vi "TipPosition.vi"(8 "error in":errorcluster) -> (0 "error out":errorcluster, 2 "CursorPosition":cluster{dbl, dbl})   [LabVIEW 2016]
uses:
  controls/Enum.ctl
  <vilib>/Utility/error.llb/Error Cluster From Error Code.vi
  <vilib>/rvi/errors/niLvFpgaAdjustHostInterfaceError.vi
  <vilib>/rvi/interface/nirviReadWriteControl/nirviReadWriteControl.xnode
  controls/FPGAVIreferenceTypeDefScanEngine.ctl
  FPGA Bitfiles/qnmController797_usbRIO_controllerFPGAmu.lvbitx
  NiFpgaLv.dll
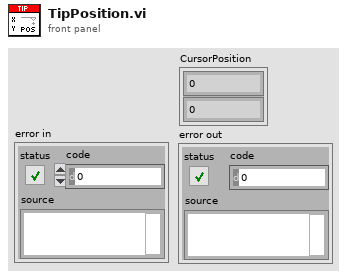
[diagram p1: front panel]
types:
  T1 = typedef "Enum.ctl" = enum16{"Init", "Read", "Write"}
  T2 = cluster{"Width":dbl, "Height":dbl, "X Offset":dbl, "Y Offset":dbl, "Angle":dbl, "Pixels/Line":u16, "Lines":u16, "Time/Line":dbl, "Scan Rate":dbl}
  T3 = cluster{"calibName":string[], "calibParameters":cluster{"Sensitivity":cluster{"Sens X":dbl, "Sens Y":dbl, "Sens Z":dbl}, "Range":cluster{"Range X":dbl, "Range Y":dbl, "Range Z":dbl}, "HV gain":cluster{"HV gain X":dbl, "HV gain Y":dbl, "HV gain Z":dbl}}[], "calibIndex":i32}
  T4 = typedef "FPGAVIreferenceTypeDefScanEngine.ctl" = refnum<k20>
  T5 = cluster{"Sensitivity":cluster{"Sens X":dbl, "Sens Y":dbl, "Sens Z":dbl}, "Range":cluster{"Range X":dbl, "Range Y":dbl, "Range Z":dbl}, "HV gain":cluster{"HV gain X":dbl, "HV gain Y":dbl, "HV gain Z":dbl}}[]
  T6 = cluster{"xOut":fxp<+/-,18,2>, "yOut":fxp<+/-,18,2>}
  T7 = cluster{"Sensitivity":cluster{"Sens X":dbl, "Sens Y":dbl, "Sens Z":dbl}, "Range":cluster{"Range X":dbl, "Range Y":dbl, "Range Z":dbl}, "HV gain":cluster{"HV gain X":dbl, "HV gain Y":dbl, "HV gain Z":dbl}}
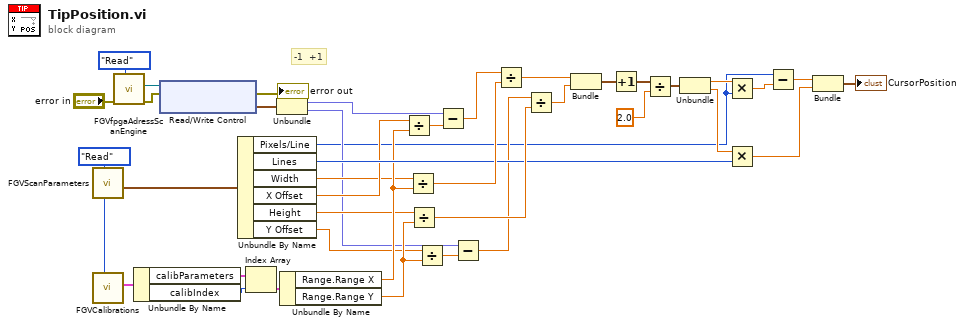
[diagram p0: block diagram]
diagram:
  w36 = Enum."Read" ("Enum")
  # "-1  +1"
  n1 = call "FGVScanParameters.vi"("Enum"=w36) -> ("Scan Parameters Out"=w35:T2)  [unwired: 9 in, 1 out]
  n2 = call "FGVCalibrations.vi"("Enum"=w36) -> ("calibOut"=w37:T3)  [unwired: 9 in, 1 out]
  n3 = call "FGVfpgaAdressScanEngine.vi"("Enum"=Enum."Read", "error in"="error in") -> ("error out"=w34:errorcluster, "FPGA.SEout"=w32:T4)  [unwired: 5 in, 3 out]
  n4 = Unbundle By Name(w37) -> ("calibParameters"=w38:T5, "calibIndex"=w39:i32)
  n5 = xnode "Read/Write Control"("FPGA VI Reference In"=w32, "error in"=w34) -> ("error out"=→"error out":errorcluster, "se.mot.s.origin"=w29:T6)  [unwired: 1 out]
  n6 = Unbundle By Name(w35) -> ("Pixels/Line"=w3:u16, "Lines"=w17:u16, "Width"=w10:dbl, "X Offset"=w13:dbl, "Height"=w9:dbl, "Y Offset"=w7:dbl)
  n7 = Index Array(array=w38, index=w39) -> (element=w40:T7)
  n8 = Unbundle(w29) -> ("xOut"=w12:fxp<+/-,18,2>, "yOut"=w6:fxp<+/-,18,2>)
  n9 = Unbundle By Name(w40) -> ("Range.Range X"=w14:dbl, "Range.Range Y"=w8:dbl)
  n10 = Divide(x=w13, y=w14) -> (x/y=w15:dbl)
  n11 = Divide(x=w10, y=w14) -> (x/y=w28:dbl)
  n12 = Divide(x=w9, y=w8) -> (x/y=w27:dbl)
  n13 = Divide(x=w7, y=w8) -> (x/y=w5:dbl)
  n14 = Subtract(x=w12, y=w15) -> (x-y=w11:dbl)
  n15 = Subtract(x=w6, y=w5) -> (x-y=w4:dbl)
  n16 = Divide(x=w11, y=w28) -> (x/y=w26:dbl)
  n17 = Divide(x=w4, y=w27) -> (x/y=w25:dbl)
  n18 = Bundle(w26, w25) -> (w24:cluster{dbl, dbl})  [unwired: 1 in]
  n19 = Increment(x=w24) -> (x+1=w23:cluster{dbl, dbl})
  n20 = Divide(x=w23, y=2.0) -> (x/y=w20:cluster{dbl, dbl})
  n21 = Unbundle(w20) -> (w19:dbl, w18:dbl)
  n22 = Multiply(x=w19, y=w3) -> (x*y=w2:dbl)
  n23 = Multiply(x=w18, y=w17) -> (x*y=w16:dbl)
  n24 = Subtract(x=w3, y=w2) -> (x-y=w1:dbl)
  n25 = Bundle(w1, w16) -> (→"CursorPosition":cluster{dbl, dbl})  [unwired: 1 in]
